vi "Get Last Substring Location.vi"(9 "offset (0)":i32, 10 "regular expression":string, 11 "string":string) -> (0 "offset past match":i32, 1 "after substring":string, 2 "match substring":string, 3 "before substring":string)   [LabVIEW 2013]
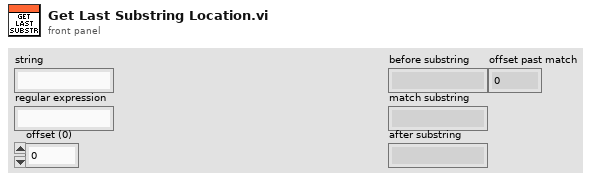
[diagram p1: front panel]
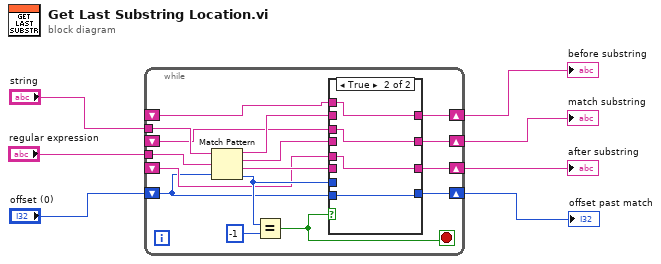
[diagram p0: block diagram]
diagram:
  n1 = while {
    tunnel: "string" -> [w23]
    tunnel: "regular expression" -> [w22]
    shift-right: [w13] -> w1
    shift-left: "offset (0)" -> [w8]
    shift-right: [w19] -> w4
    shift-left: _ -> [w11]
    shift-right: [w17] -> w3
    shift-left: _ -> [w10]
    shift-right: [w15] -> w2
    shift-left: _ -> [w9]
    stop <- w12 stop-if-true
    n2 = Match Pattern(string=w23, regular expression=w22, offset (0)=w8) -> (before substring=w20:string, match substring=w18:string, after substring=w16:string, offset past match=w14:i32)
    n3 = Equal?(x=w14, y=-1) -> (x = y?=w12:bool)
    n4 = case shown="True" w12 {
      tunnel: w20 -> [w27 _]
      tunnel: [w27 w31] -> w19
      tunnel: w18 -> [w26 _]
      tunnel: [w26 w30] -> w17
      tunnel: w16 -> [w25 _]
      tunnel: [w25 w29] -> w15
      tunnel: w14 -> [w24 _]
      tunnel: [w24 w28] -> w13
      tunnel: w11 -> [_ w31]
      tunnel: w10 -> [_ w30]
      tunnel: w9 -> [_ w29]
      tunnel: w8 -> [_ w28]
      frame False {
      }
      frame True {
      }
    }
  }
  "before substring" <- w4
  "match substring" <- w3
  "after substring" <- w2
  "offset past match" <- w1
